vi "double-get sum.vi"(8 "error in (no error)":errorcluster, 11 "(a, b) in":T1) -> (0 "error out":errorcluster, 2 "sum = a+b":i32, 3 "(a, b) out (duplicate)":T1)   [LabVIEW 2021, in "Project Euler.lvlib"]
uses:
  Project Euler.lvlib
  cluster-double.ctl
panel:
  # "Development\ncontrols/indicators useful for development and testing, but which are not outputs of the VI"
  # "Input\nInputs to the VI"
  # "Output\nOutputs of the VI"
  # "Description\n\nBlank VI with error handling case. \n\nSummarize the use of this VI in this space."
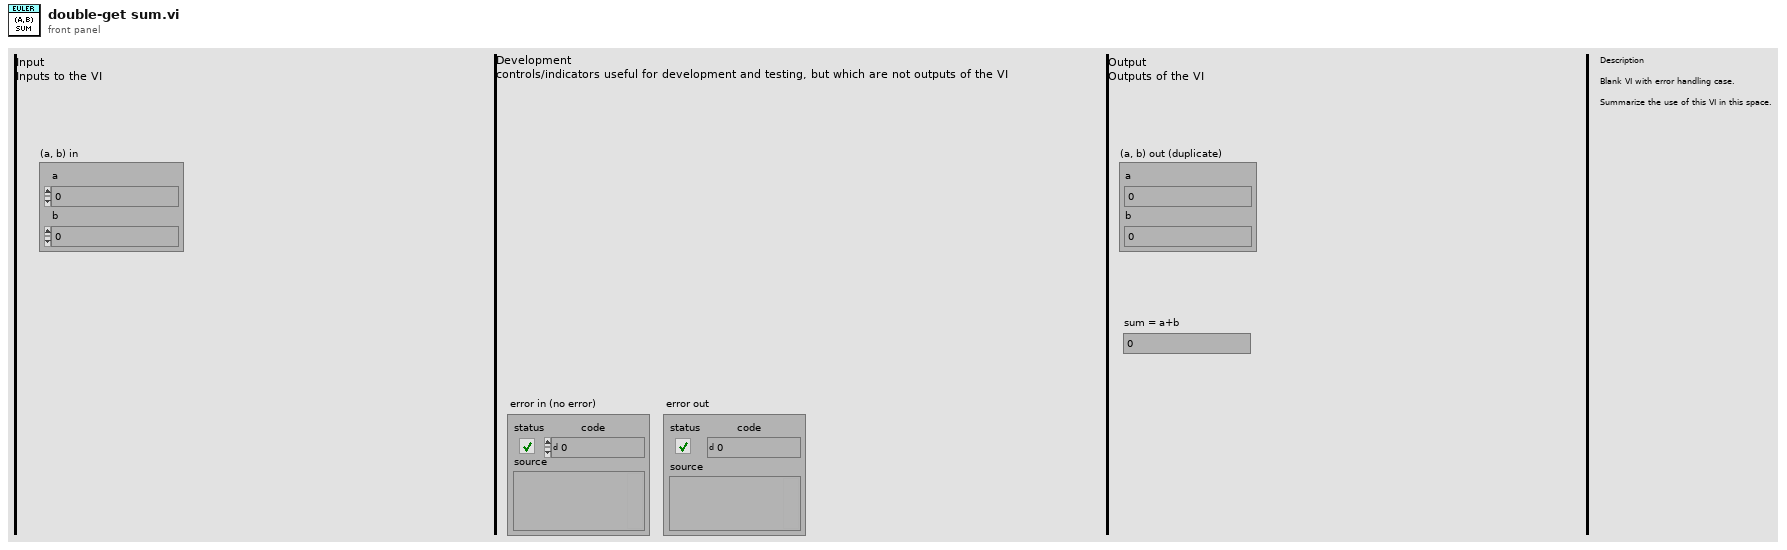
[diagram p1: front panel]
types:
  T1 = typedef "Project Euler.lvlib/cluster-double.ctl" = cluster{"a":i32, "b":i32}
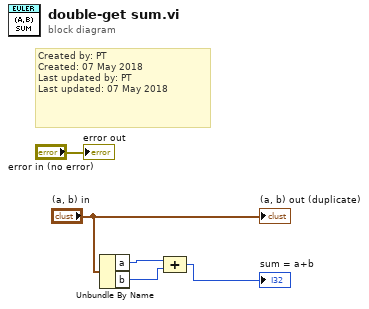
[diagram p0: block diagram]
diagram:
  # "Created by: PT\nCreated: 07 May 2018\nLast updated by: PT\nLast updated: 07 May 2018"
  n1 = Unbundle By Name("(a, b) in") -> ("a"=w3:i32, "b"=w2:i32)
  n2 = Compound Arithmetic op=ADD(w3, w2) -> (→"sum = a+b":i32)
  "error out" <- "error in (no error)"
  "(a, b) out (duplicate)" <- "(a, b) in"
